vi "Set panes to origin.vi"(8 "error in (no error)":errorcluster, 11 "Pane refs array":refnum<vi>[](array[refnum])) -> (0 "error out":errorcluster)   [LabVIEW 2013]
uses:
  <vilib>/Utility/miscctls.llb/LVPointTypeDef.ctl
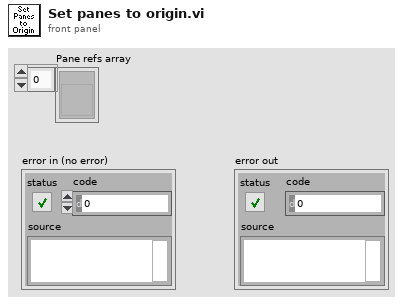
[diagram p1: front panel]
types:
  T1 = typedef "LVPointTypeDef.ctl" = cluster{"Horizontal":i16, "Vertical":i16}
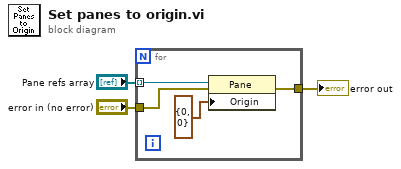
[diagram p0: block diagram]
diagram:
  n1 = for {
    tunnel: "Pane refs array" -> [w6] mode=indexing
    tunnel: [w5] -> w1
    tunnel: "error in (no error)" -> [w4]
    n2 = property class="Pane"(reference=w6, error in=w4, "Origin"=T1 {"Horizontal"=0, "Vertical"=0}) -> (error out=w5:errorcluster)  [unwired: 1 out]
  }
  "error out" <- w1
